vi "toXml.vi"(8 "error in (no error)":errorcluster, 11 "PlayFile in":refnum<class "PlayFile.lvclass">) -> (0 "error out":errorcluster, 2 "scriptEventXML":refnum<class "xmlNode.lvclass">, 3 "PlayFile out":refnum<class "PlayFile.lvclass">)   [LabVIEW 2011, in "Tools.lvlib" / "Scripting.lvlib" / "PlayFile.lvclass"]
uses:
  PlayFile.lvclass
  xmlNode/xmlNode.lvclass
  DatabaseHelpers/Database Objects/Channel/Channel.lvclass
  ScriptEvent.lvclass
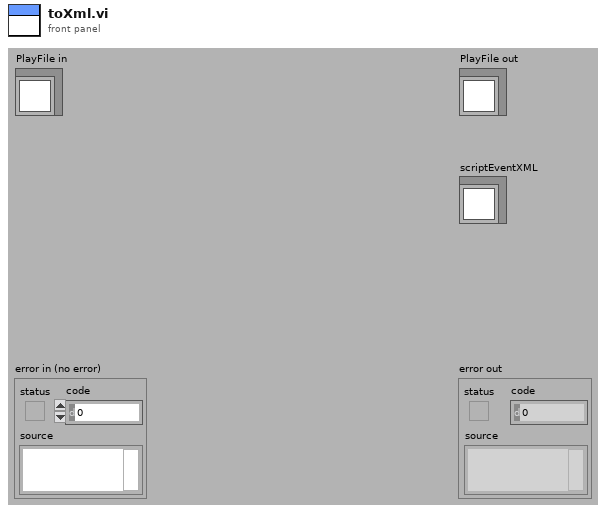
[diagram p1: front panel]
types:
  T1 = cluster{"attributeName":string, "channel_name":string}
  T2 = cluster{"attributeName":string, "channel_name":string}[]
  T3 = cluster{"parameter_name":string, "parameter_value":string, "type":enum16{"time", "time_difference", "value", "frequency", "phase", "ramp_time", "value_step", "time_step", "number_of_steps", "start_value", "end_value", "start_freq", "start_amp", "start_phase", "end_freq", "end_amp", "end_phase"}}[]
  T4 = enum16{"time", "time_difference", "value", "frequency", "phase", "ramp_time", "value_step", "time_step", "number_of_steps", "start_value", "end_value", "start_freq", "start_amp", "start_phase", "end_freq", "end_amp", "end_phase"}
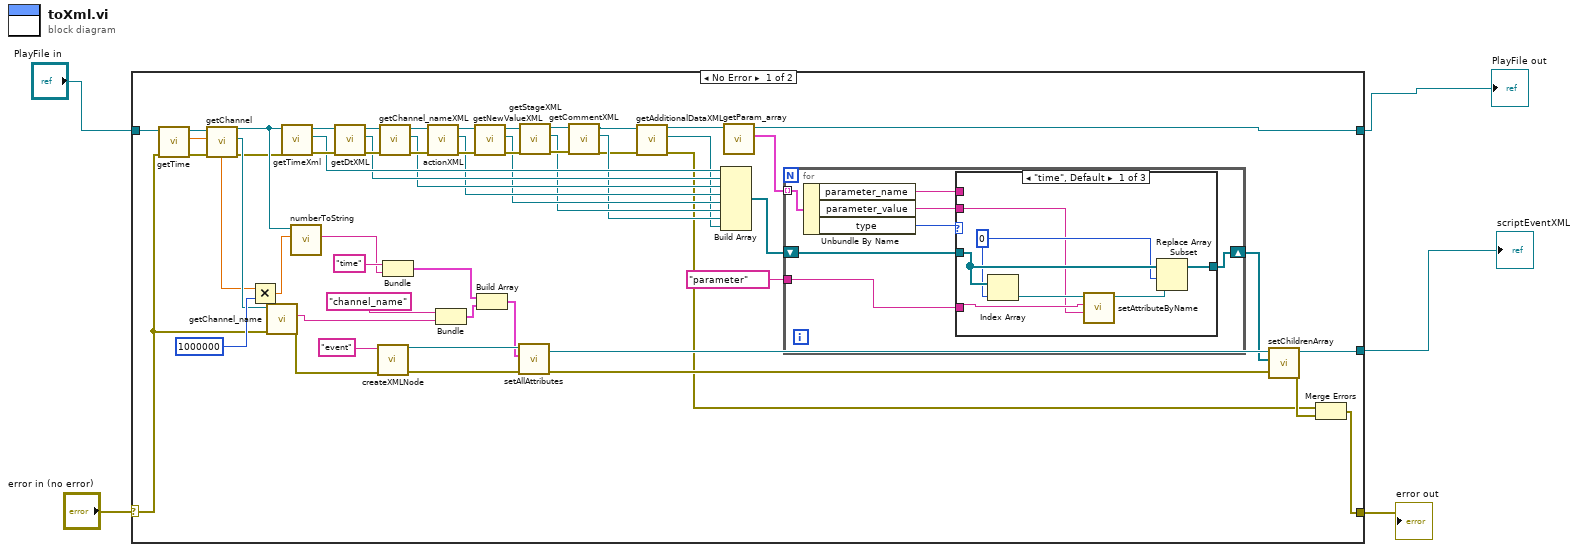
[diagram p0: block diagram]
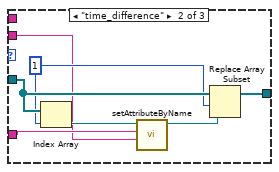
[diagram p2: hidden frame]
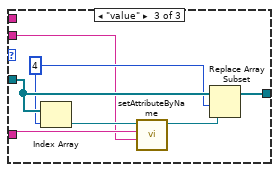
[diagram p3: hidden frame]
diagram:
  n1 = case shown="No Error" "error in (no error)" {
    selector: "error in (no error)" -> [w16 w90]
    tunnel: [w38 w90] -> w1
    tunnel: [w8 w89] -> w3
    tunnel: "PlayFile in" -> [w22 w89]
    tunnel: [w24 _] -> w2
    frame No Error {
      n2 = call "getTime.vi"("error in (no error)"=w16, "ScriptEvent.lvclass in"=w22) -> ("error out"=w17:errorcluster, "time"=w19:dbl, "ScriptEvent.lvclass out"=w23:refnum<class "PlayFile.lvclass">)  [unwired: 7 in]
      n3 = call-dynamic "getChannel.vi"("error in (no error)"=w17, "ScriptEvent.lvclass in"=w23) -> ("error out"=w18:errorcluster, "Channel.lvclass"=w20:refnum<class "Channel.lvclass">, "ScriptEvent.lvclass out"=w21:refnum<class "PlayFile.lvclass">)  [unwired: 7 in]
      n4 = Multiply(x=w19, y=1000000) -> (x*y=w26:dbl)
      n5 = call "getChannel_name.vi"("error in (no error)"=w16, "Channel.lvclass in"=w20) -> ("error out"=w59:errorcluster, "channel_name"=w35:string)  [unwired: 7 in, 1 out]
      n6 = call "getTimeXml.vi"("error in (no error)"=w18, "ScriptEvent in"=w21) -> ("error out"=w58:errorcluster, "timeXML"=w46:refnum<class "xmlNode.lvclass">, "ScriptEvent out"=w52:refnum<class "PlayFile.lvclass">)  [unwired: 7 in]
      n7 = call "numberToString.vi"("Numeric"=w26, "ScriptEvent in"=w21) -> ("String"=w25:string)  [unwired: 7 in, 2 out]
      n8 = call "getDtXML.vi"("error in (no error)"=w58, "ScriptEvent in"=w52) -> ("error out"=w57:errorcluster, "dtXML"=w45:refnum<class "xmlNode.lvclass">, "ScriptEvent out"=w51:refnum<class "PlayFile.lvclass">)  [unwired: 7 in]
      n9 = call "createXMLNode.vi"("error in (no error)"=w59, "name"="event") -> ("error out"=w30:errorcluster, "xmlNode out"=w34:refnum<class "xmlNode.lvclass">)  [unwired: 8 in]
      n10 = call "getChannel_nameXML.vi"("error in (no error)"=w57, "ScriptEvent in"=w51) -> ("error out"=w56:errorcluster, "channel_nameXML"=w44:refnum<class "xmlNode.lvclass">, "ScriptEvent out"=w50:refnum<class "PlayFile.lvclass">)  [unwired: 7 in]
      n11 = Bundle("attributeName"="time", "String"=w25) -> (w33:cluster{"attributeName":string, "String":string})  [unwired: 1 in]
      n12 = call "actionXML.vi"("error in (no error)"=w56, "ScriptEvent in"=w50) -> ("error out"=w55:errorcluster, "actionXml"=w43:refnum<class "xmlNode.lvclass">, "ScriptEvent out"=w49:refnum<class "PlayFile.lvclass">)  [unwired: 7 in]
      n13 = Bundle("attributeName"="channel_name", "channel_name"=w35) -> (w32:T1)  [unwired: 1 in]
      n14 = call-dynamic "getNewValueXML.vi"("error in (no error)"=w55, "ScriptEvent in"=w49) -> ("error out"=w54:errorcluster, "newValueXML"=w42:refnum<class "xmlNode.lvclass">, "ScriptEvent out"=w48:refnum<class "PlayFile.lvclass">)  [unwired: 7 in]
      n15 = Build Array(w33, w32) -> (w31:T2)
      n16 = call-dynamic "setAllAttributes.vi"("error in (no error)"=w30, "attributes"=w31, "xmlNode in"=w34) -> ("error out"=w29:errorcluster, "xmlNode out"=w28:refnum<class "xmlNode.lvclass">)  [unwired: 7 in]
      n17 = call "getStageXML.vi"("error in (no error)"=w54, "ScriptEvent in"=w48) -> ("error out"=w53:errorcluster, "stageXML"=w41:refnum<class "xmlNode.lvclass">, "ScriptEvent out"=w47:refnum<class "PlayFile.lvclass">)  [unwired: 7 in]
      n18 = call "getCommentXML.vi"("error in (no error)"=w53, "ScriptEvent in"=w47) -> ("error out"=w14:errorcluster, "commentXML"=w40:refnum<class "xmlNode.lvclass">, "ScriptEvent out"=w15:refnum<class "PlayFile.lvclass">)  [unwired: 7 in]
      n19 = call-dynamic "getAdditionalDataXML.vi"("error in (no error)"=w14, "PlayFile in"=w15) -> ("error out"=w13:errorcluster, "additionalDataXML"=w12:refnum<class "xmlNode.lvclass">, "PlayFile out"=w9:refnum<class "PlayFile.lvclass">)  [unwired: 7 in]
      n20 = Build Array(w46, w45, w44, w43, w42, w41, w40, w12) -> (w7:refnum<class "xmlNode.lvclass">[])
      n21 = call "getParam_array.vi"("ScriptEvent in"=w9) -> ("param_array"=w11:T3, "ScriptEvent out"=w8:refnum<class "PlayFile.lvclass">)  [unwired: 8 in, 1 out]
      n22 = for {
        tunnel: w11 -> [w67] mode=indexing
        shift-right: [w62] -> w6
        shift-left: w7 -> [w65]
        tunnel: "parameter" -> [w61]
        n23 = Unbundle By Name(w67) -> ("parameter_name"=w64:string, "parameter_value"=w63:string, "type"=w66:T4)
        n24 = case shown="\"time\", Default" w66 {
          tunnel: w65 -> [w72 w79 w86]
          tunnel: w64 -> [_ _ _]
          tunnel: w63 -> [w68 w75 w82]
          tunnel: [w70 w77 w84] -> w62
          tunnel: w61 -> [w69 w76 w83]
          frame "time", Default {
            w71 = 0
            n25 = Index Array(array=w72, index=w71) -> (element=w74:refnum<class "xmlNode.lvclass">)
            n26 = call-dynamic "setAttributeByName.vi"("attributeValue"=w68, "attributeName"=w69, "xmlNode in"=w74) -> ("xmlNode out"=w73:refnum<class "xmlNode.lvclass">)  [unwired: 7 in, 1 out]
            n27 = Replace Array Subset(array=w72, new element=w73, index=w71) -> (w70:refnum<class "xmlNode.lvclass">[])
          }
          frame "time_difference" {
            w78 = 1
            n28 = Index Array(array=w79, index=w78) -> (element=w81:refnum<class "xmlNode.lvclass">)
            n29 = call-dynamic "setAttributeByName.vi"("attributeValue"=w75, "attributeName"=w76, "xmlNode in"=w81) -> ("xmlNode out"=w80:refnum<class "xmlNode.lvclass">)  [unwired: 7 in, 1 out]
            n30 = Replace Array Subset(array=w79, new element=w80, index=w78) -> (w77:refnum<class "xmlNode.lvclass">[])
          }
          frame "value" {
            w85 = 4
            n31 = Index Array(array=w86, index=w85) -> (element=w88:refnum<class "xmlNode.lvclass">)
            n32 = call-dynamic "setAttributeByName.vi"("attributeValue"=w82, "attributeName"=w83, "xmlNode in"=w88) -> ("xmlNode out"=w87:refnum<class "xmlNode.lvclass">)  [unwired: 7 in, 1 out]
            n33 = Replace Array Subset(array=w86, new element=w87, index=w85) -> (w84:refnum<class "xmlNode.lvclass">[])
          }
        }
      }
      n34 = call-dynamic "setChildrenArray.vi"("error in (no error)"=w29, "Children"=w6, "xmlNode.lvclass in"=w28) -> ("error out"=w39:errorcluster, "xmlNode.lvclass out"=w24:refnum<class "xmlNode.lvclass">)  [unwired: 7 in]
      n35 = Merge Errors(w13, w39) -> (w38:errorcluster)
    }
    frame Error {
    }
  }
  "error out" <- w1
  "PlayFile out" <- w3
  "scriptEventXML" <- w2
